vi "读取数据库.vi"(6 "精度(6)":i16=2, 7 "condition":string, 8 "error in (no error)":errorcluster caption="错误输入（无错误）", 9 "database":string="database1.mdb", 10 "显示项":string[](array[string]), 11 "组合框":string(combo)) -> (0 "error out":errorcluster caption="错误输出", 1 "columns":string[](array[string]), 2 "data":variant[][](array[variant]), 3 "表格":string[][](table))   [LabVIEW 2016]
uses:
  <vilib>/Utility/sysdir.llb/System Directory Type.ctl
  <vilib>/addons/database/Connection.llb/DB Tools Open Connec (String).vi
  <vilib>/addons/database/_DB Variant To Data/Database Variant To Data.xnode
  <vilib>/addons/database/NI_Database_API.lvlib
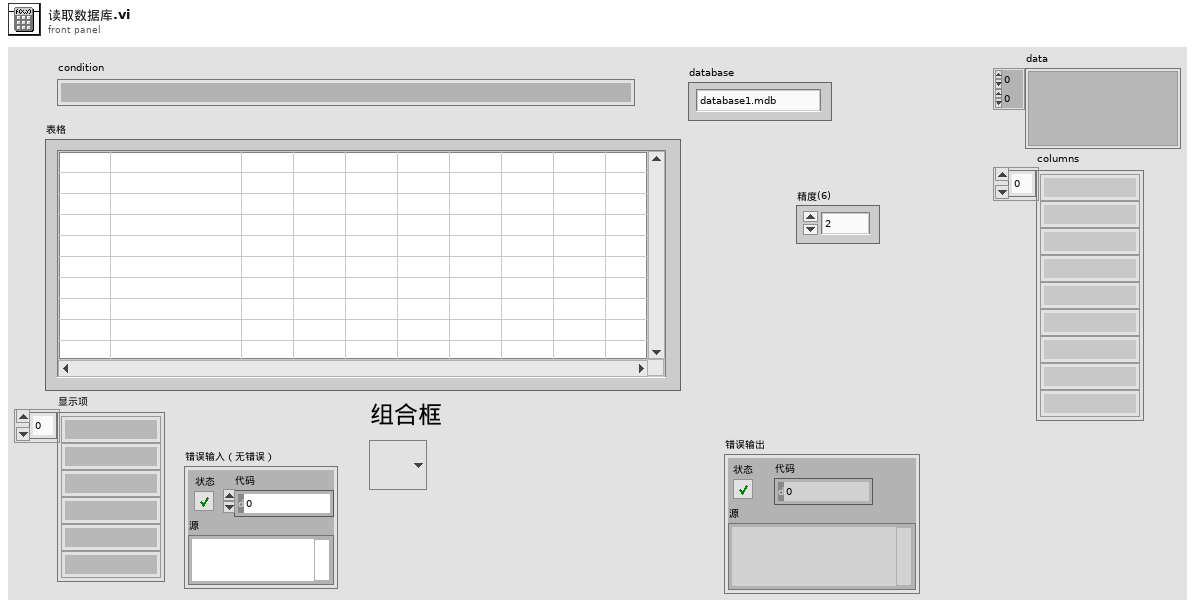
[diagram p1: front panel]
types:
  T1 = typedef "System Directory Type.ctl" = i32
  T2 = typedef "NI_Database_API.lvlib/Conn ObjectReference.ctl" = refnum<k1>
  T3 = typedef "NI_Database_API.lvlib/DB Tools DataTypes.ctl" = enum16{"String", "Long (I32)", "Single (SGL)", "Double (DBL)", "Date/Time", "Binary"}
  T4 = cluster{"name":string, "database data type":T3, "defined size":i32}[]
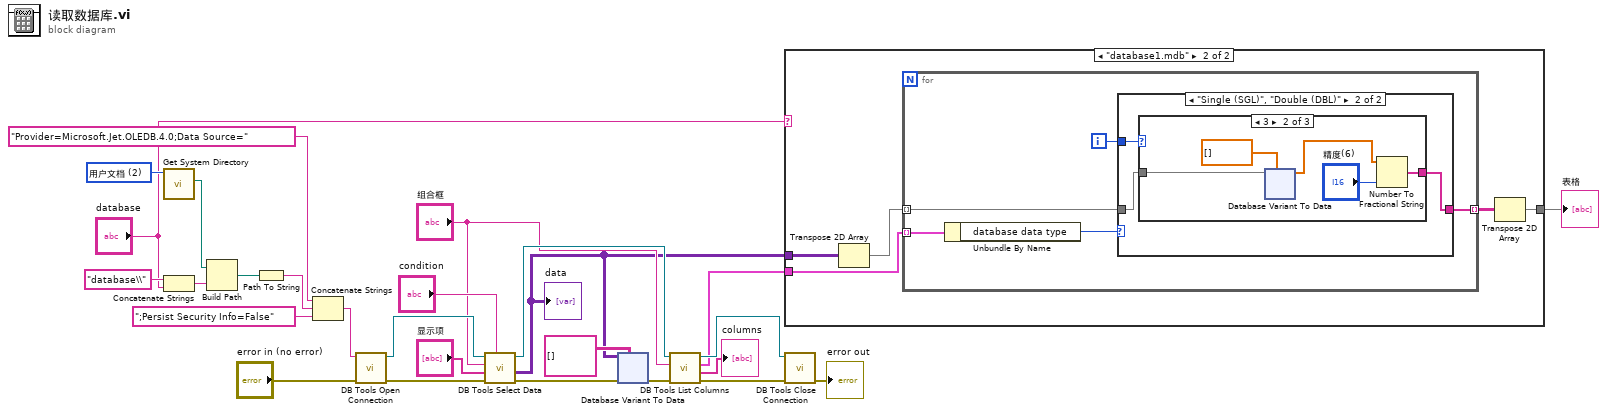
[diagram p0: block diagram]
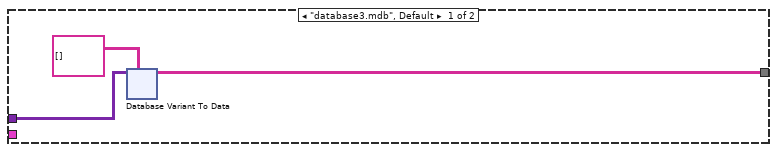
[diagram p2: hidden frame]
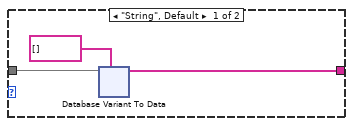
[diagram p3: hidden frame]
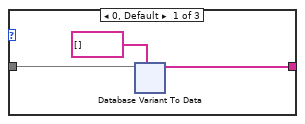
[diagram p4: hidden frame]
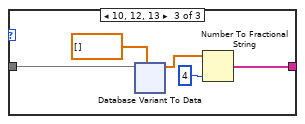
[diagram p5: hidden frame]
diagram:
  w11 = T1 2 items=["用户目录"=0, "用户桌面"=1, "用户文档"=2, "用户应用程序数据"=3, "用户设置"=4, "用户临时目录"=5, "公共文档"=6, "公共应用程序数据"=7, "公共设置"=8, "公共缓存"=13, "系统核心库"=9, "系统安装库"=10, "应用程序文件"=11, "启动盘根目录"=12] ("system directory type")
  n1 = call <vilib>:"Get System Directory.vi"("system directory type"=w11) -> ("system directory"=w10:path)  [unwired: 10 in]
  n2 = Concatenate Strings("database\\" ("名称或相对路径"), "database") -> (w6:string)
  n3 = Build Path(base path=w10, name or relative path=w6) -> (appended path=w12:path)
  n4 = Path To String(path=w12) -> (string=w13:string)
  n5 = Concatenate Strings("Provider=Microsoft.Jet.OLEDB.4.0;Data Source=", w13, ";Persist Security Info=False") -> (w9:string)
  n6 = call-poly <vilib>:"DB Tools Open Connection.vi"("error in (no error)"="error in (no error)", "connection information"=w9) -> ("error out"=w26:errorcluster, "connection reference"=w27:T2)  [unwired: 6 in]
  n7 = call <vilib>:"DB Tools Select Data.vi"("condition"="condition", "error in (no error)"=w26, "columns"="显示项", "table"="组合框", "connection reference"=w27) -> ("error out"=w25:errorcluster, "data"=w3:variant[][], "connection reference out"=w20:T2)  [unwired: 1 in]
  "data" <- w3
  n8 = xnode "Database Variant To Data"("database variant"=w3, "error in (no error)"=w25, "type"=string[][] []) -> ("error out"=w21:errorcluster)  [unwired: 1 out]
  n9 = call <vilib>:"DB Tools List Columns.vi"("error in (no error)"=w21, "table"="组合框", "connection reference"=w20) -> ("error out"=w16:errorcluster, "columns"=→"columns":string[], "column information"=w2:T4, "connection reference out"=w17:T2)  [unwired: 1 in]
  n10 = case shown="\"database1.mdb\"" "database" {
    tunnel: w3 -> [w29 w79]
    tunnel: w2 -> [_ w77]
    tunnel: [w28 w75] -> w1
    frame "database3.mdb", Default {
      n11 = xnode "Database Variant To Data"("database variant"=w29, "type"=string[][] []) -> ("data"=w28:string[][])  [unwired: 1 in, 1 out]
    }
    frame "database1.mdb" {
      n12 = Transpose 2D Array(2D array=w79) -> (transposed array=w78:variant[][])
      n13 = for {
        tunnel: w78 -> [w82] mode=indexing
        tunnel: w77 -> [w84] mode=indexing
        tunnel: [w81] -> w76 mode=indexing
        i -> [w80]
        n14 = Unbundle By Name(w84) -> ("database data type"=w83:T3)
        n15 = case shown="\"Single (SGL)\", \"Double (DBL)\"" w83 {
          tunnel: w82 -> [w86 w128]
          tunnel: [w85 w127] -> w81
          tunnel: w80 -> [_ w126]
          frame "String", Default {
            n16 = xnode "Database Variant To Data"("database variant"=w86, "type"=string[] []) -> ("data"=w85:string[])  [unwired: 1 in, 1 out]
          }
          frame "Single (SGL)", "Double (DBL)" {
            n17 = case shown="3" w126 {
              tunnel: w128 -> [w130 w174 w214]
              tunnel: [w129 w170 w215] -> w127
              frame 0, Default {
                n18 = xnode "Database Variant To Data"("database variant"=w130, "type"=string[] []) -> ("data"=w129:string[])  [unwired: 1 in, 1 out]
              }
              frame 3 {
                n19 = xnode "Database Variant To Data"("database variant"=w174, "type"=dbl[] []) -> ("data"=w172:dbl[])  [unwired: 1 in, 1 out]
                n20 = Number To Fractional String(number=w172, precision (6)="精度(6)") -> (F-format string=w170:string[])  [unwired: 2 in]
              }
              frame 10, 12, 13 {
                n21 = xnode "Database Variant To Data"("database variant"=w214, "type"=dbl[] []) -> ("data"=w213:dbl[])  [unwired: 1 in, 1 out]
                n22 = Number To Fractional String(number=w213, precision (6)=i16 4 ("精度(6)")) -> (F-format string=w215:string[])  [unwired: 2 in]
              }
            }
          }
        }
      }
      n23 = Transpose 2D Array(2D array=w76) -> (transposed array=w75:string[][])
    }
  }
  "表格" <- w1
  n24 = call <vilib>:"DB Tools Close Connection.vi"("error in (no error)"=w16, "connection reference"=w17) -> ("error out"=→"error out":errorcluster)  [unwired: 5 in]
